vi "uTTA_TestFileUpload.vi"() -> ()   [LabVIEW 2021]
panel:
  out "error out":errorcluster
  in  "File Path":path
  out "Identity":string
  in  "VISA in":refnum<visa-resource-name>
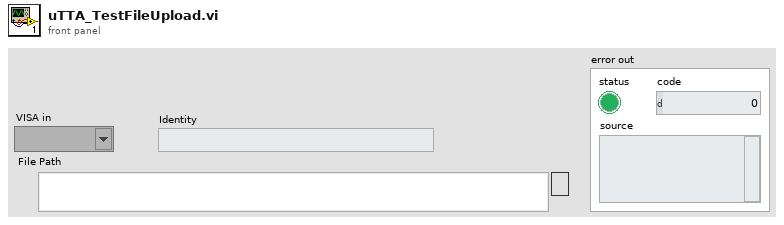
[diagram p1: front panel]
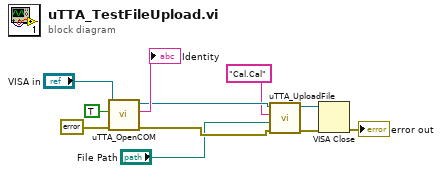
[diagram p0: block diagram]
diagram:
  n1 = call "uTTA_OpenCOM.vi"("error in"=errorcluster {"status"=FALSE, "code"=0, "source"=""}, "Log Serial Monitor(T)"=TRUE ("Log Serial Monitor"), "VISA in"="VISA in") -> ("error out"=w6:errorcluster, "Identity"=→"Identity":string, "VISA out"=w7:refnum<visa-resource-name>)  [unwired: 6 in]
  n2 = call "uTTA_UploadFile.vi"("error in"=w6, "File Path"="File Path", "File Name"="Cal.Cal", "VISA Refnum in"=w7) -> ("error out"=w3:errorcluster, "VISA Refnum out"=w2:refnum<visa-resource-name>)  [unwired: 6 in]
  n3 = VISA Close(VISA resource name=w2, error in (no error)=w3) -> (error out=→"error out":errorcluster)
